vi "treadmill_main.vi"() -> ()   [LabVIEW 2019]
uses:
  #typedef_DefinedStates.ctl
  OperateCluster.ctl
  SpeedAndTimeCluster.ctl
  FollowingSteps.ctl
panel:
  out "Speed":u16
  out "Time":dbl
  in  "Slower":bool
  in  "Faster":bool
  in  "Exit":bool
  in  "QuickStart":bool
  in  "Start Program":bool
  in  "DefineProg":bool
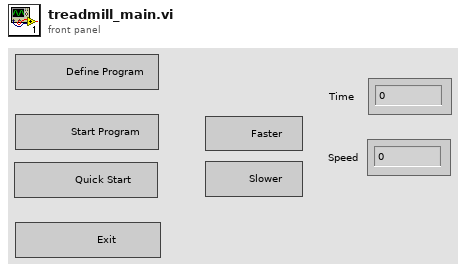
[diagram p1: front panel]
types:
  T1 = typedef "OperateCluster.ctl" = cluster{"SpeedAndTime":T2, "Following Steps":T3, "CurrentStep 2":T2, "WorkStepsCoutner":u16, "LastIndex":i32, "LastState":T4}
  T2 = typedef "SpeedAndTimeCluster.ctl" = cluster{"Time ":dbl, " Speed":u16}
  T3 = typedef "FollowingSteps.ctl" = T2[]
  T4 = typedef "#typedef_DefinedStates.ctl" = enum16{"Init", "Config", "DefineProgram", "StartProgram", "WorkAsUWant", "ChangeStep", "WorkwithSteps", "ExitProgram"}
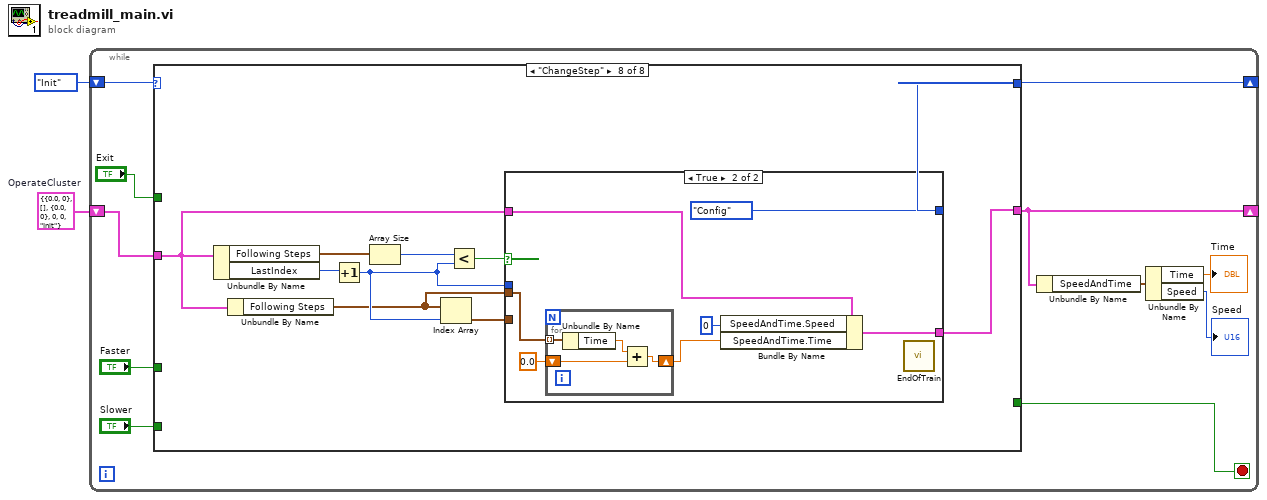
[diagram p0: block diagram]
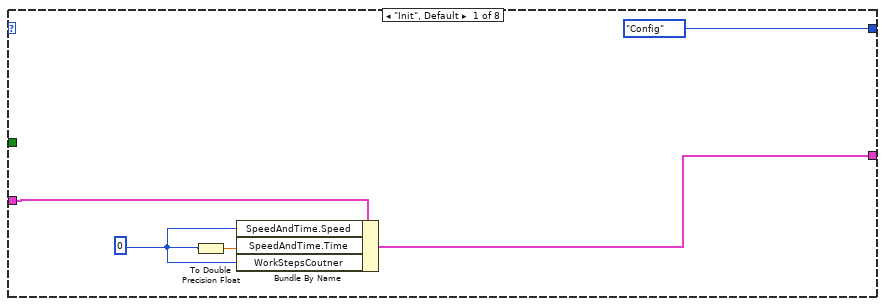
[diagram p2: hidden frame]
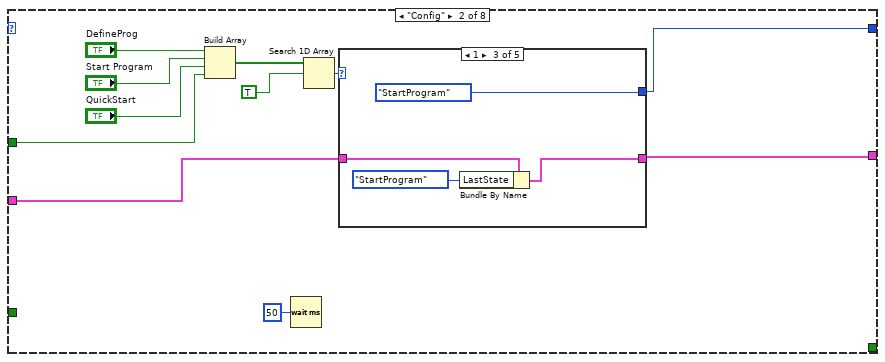
[diagram p3: hidden frame]
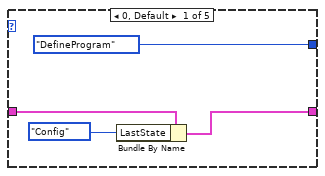
[diagram p4: hidden frame]
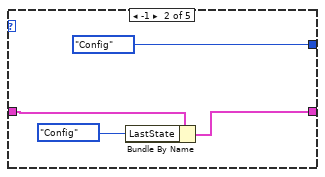
[diagram p5: hidden frame]
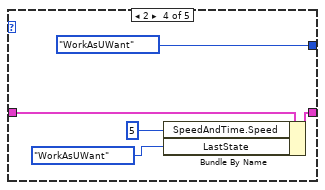
[diagram p6: hidden frame]
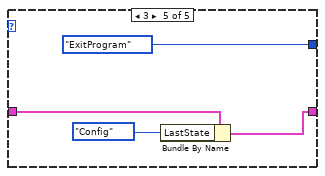
[diagram p7: hidden frame]
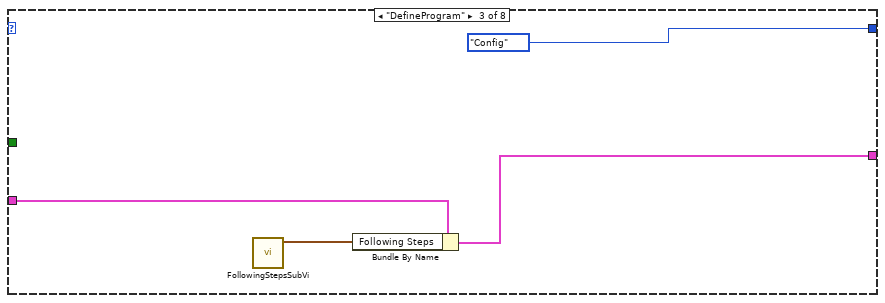
[diagram p8: hidden frame]
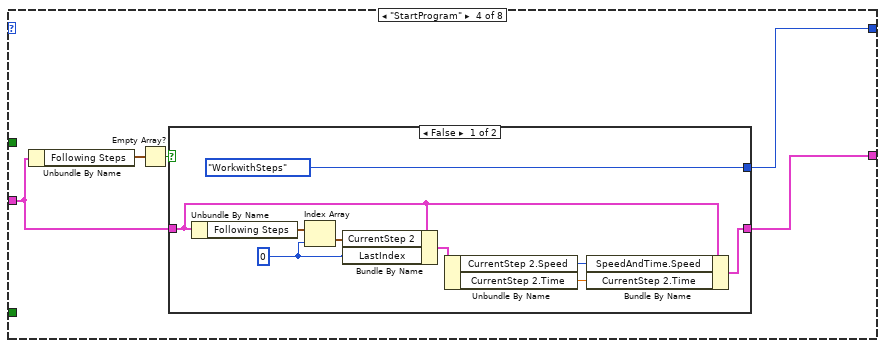
[diagram p9: hidden frame]
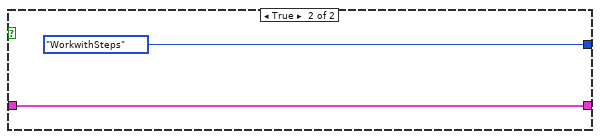
[diagram p10: hidden frame]
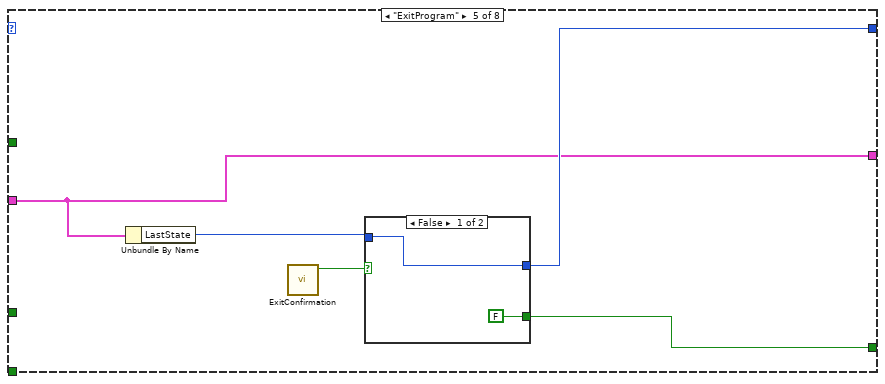
[diagram p11: hidden frame]
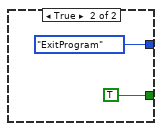
[diagram p12: hidden frame]
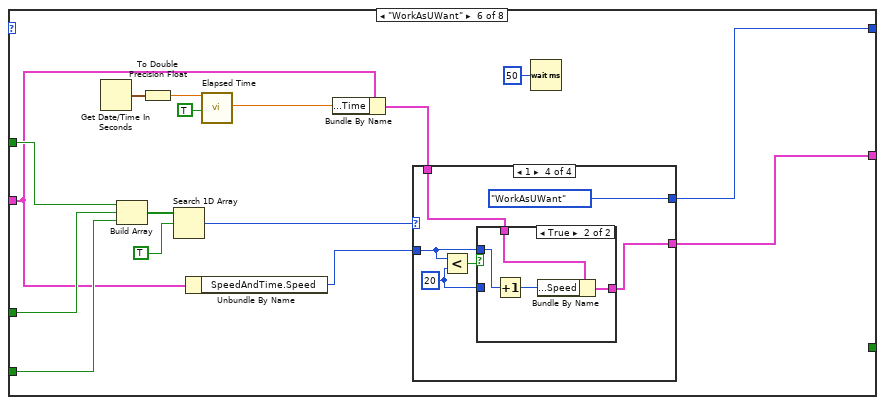
[diagram p13: hidden frame]
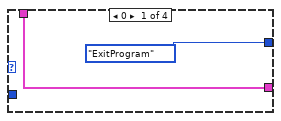
[diagram p14: hidden frame]
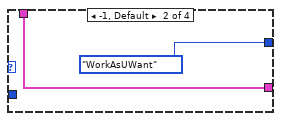
[diagram p15: hidden frame]
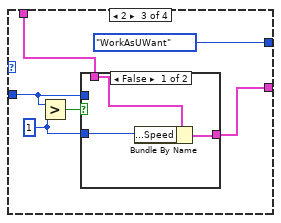
[diagram p16: hidden frame]
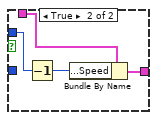
[diagram p17: hidden frame]
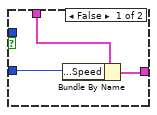
[diagram p18: hidden frame]
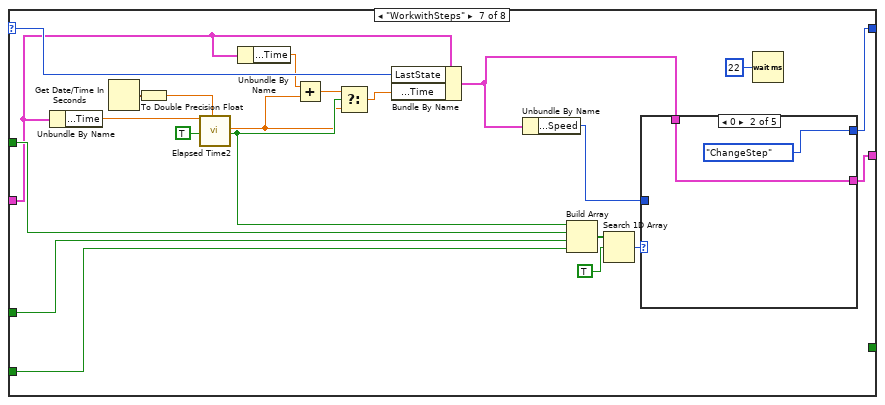
[diagram p19: hidden frame]
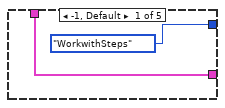
[diagram p20: hidden frame]
diagram:
  w1 = T1 {"SpeedAndTime"={"Time "=0.0, " Speed"=0}, "Following Steps"=[], "CurrentStep 2"={"Time "=0.0, " Speed"=0}, "WorkStepsCoutner"=0, "LastIndex"=0, "LastState"=enum."Init"}  # OperateCluster
  n1 = while {
    shift-right: [w11] -> _
    shift-left: #typedef_DefinedStates."Init" -> [w3]
    shift-right: [w9] -> _
    shift-left: w1 -> [w10]
    stop <- w4 stop-if-true
    n2 = case shown="\"ChangeStep\"" w3 {
      selector: w3 -> [_ _ _ _ _ _ w137 _]
      tunnel: [#typedef_DefinedStates."Config" w21 #typedef_DefinedStates."Config" w57 w74 w89 w138 w181] -> w11
      tunnel: w10 -> [w17 w24 w52 w56 w72 w86 w131 w184]
      tunnel: [w16 w23 w51 w55 w72 w88 w139 w186] -> w9
      tunnel: "Faster" -> [_ _ _ _ _ w95 w143 _]
      tunnel: "Slower" -> [_ _ _ _ _ w94 w144 _]
      tunnel: "Exit" -> [_ w20 _ _ _ w90 w142 _]
      tunnel: [_ _ _ _ w73 _ _ _] -> w4
      frame "Init", Default {
        w14 = u16 0 ("index")
        n3 = To Double Precision Float(number=w14) -> (double precision float=w15:dbl)
        n4 = Bundle By Name(cluster=w17, "SpeedAndTime.Speed"=w14, "SpeedAndTime.Time"=w15, "WorkStepsCoutner"=w14) -> (w16:T1)
      }
      frame "Config" {
        n5 = Build Array("DefineProg", "Start Program", "QuickStart", w20) -> (w26:bool[])
        n6 = Wait (ms)(milliseconds to wait=u32 50) -> ()  [unwired: 1 out]
        n7 = Search 1D Array(1D array=w26, element=TRUE) -> (index of element=w25:i32)  [unwired: 1 in]
        n8 = case shown="1" w25 {
          tunnel: [#typedef_DefinedStates."DefineProgram" #typedef_DefinedStates."Config" #typedef_DefinedStates."StartProgram" #typedef_DefinedStates."WorkAsUWant" #typedef_DefinedStates."ExitProgram"] -> w21
          tunnel: w24 -> [w32 w35 w39 w46 w48]
          tunnel: [w31 w34 w38 w45 w47] -> w23
          frame 0, Default {
            n9 = Bundle By Name(cluster=w32, "LastState"=#typedef_DefinedStates."Config") -> (w31:T1)
          }
          frame -1 {
            n10 = Bundle By Name(cluster=w35, "LastState"=#typedef_DefinedStates."Config") -> (w34:T1)
          }
          frame 1 {
            n11 = Bundle By Name(cluster=w39, "LastState"=#typedef_DefinedStates."StartProgram") -> (w38:T1)
          }
          frame 2 {
            n12 = Bundle By Name(cluster=w46, "SpeedAndTime.Speed"=u16 5 ("CurrentStep 2. Speed"), "LastState"=#typedef_DefinedStates."WorkAsUWant") -> (w45:T1)
          }
          frame 3 {
            n13 = Bundle By Name(cluster=w48, "LastState"=#typedef_DefinedStates."Config") -> (w47:T1)
          }
        }
      }
      frame "DefineProgram" {
        n14 = call "FollowingStepsSubVi.vi"() -> ("ArrayOutput"=w53:T3)  [unwired: 11 in]
        n15 = Bundle By Name(cluster=w52, "Following Steps"=w53) -> (w51:T1)
      }
      frame "StartProgram" {
        n16 = Unbundle By Name(w56) -> ("Following Steps"=w59:T3)
        n17 = Empty Array?(array=w59) -> (empty?=w58:bool)
        n18 = case shown="False" w58 {
          tunnel: [#typedef_DefinedStates."WorkwithSteps" #typedef_DefinedStates."WorkwithSteps"] -> w57
          tunnel: w56 -> [w63 w69]
          tunnel: [w62 w69] -> w55
          frame False {
            w65 = 0 ("index")
            n19 = Unbundle By Name(w63) -> ("Following Steps"=w67:T3)
            n20 = Index Array(array=w67, index=w65) -> (element=w66:T2)
            n21 = Bundle By Name(cluster=w63, "CurrentStep 2"=w66, "LastIndex"=w65) -> (w64:T1)
            n22 = Unbundle By Name(w64) -> ("CurrentStep 2.Speed"=w61:u16, "CurrentStep 2.Time"=w60:dbl)
            n23 = Bundle By Name(cluster=w63, "SpeedAndTime.Speed"=w61, "CurrentStep 2.Time"=w60) -> (w62:T1)
          }
          frame True {
          }
        }
      }
      frame "ExitProgram" {
        n24 = Unbundle By Name(w72) -> ("LastState"=w71:T4)
        n25 = call "ExitConfirmation.vi"() -> ("Output"=w75:bool)  [unwired: 11 in]
        n26 = case shown="False" w75 {
          tunnel: [w77 #typedef_DefinedStates."ExitProgram"] -> w74
          tunnel: [FALSE TRUE] -> w73
          tunnel: w71 -> [w77 _]
          frame False {
          }
          frame True {
          }
        }
      }
      frame "WorkAsUWant" {
        n27 = Get Date/Time In Seconds() -> (seconds since 1Jan1904=w84:timestamp)
        n28 = Build Array(w90, w95, w94) -> (w93:bool[])
        n29 = To Double Precision Float(number=w84) -> (double precision float=w81:dbl)
        n30 = Search 1D Array(1D array=w93, element=TRUE) -> (index of element=w91:i32)  [unwired: 1 in]
        n31 = Unbundle By Name(w86) -> ("SpeedAndTime.Speed"=w87:u16)
        n32 = call "Elapsed Time"("Time Target (s)"=w81, "Auto Reset"=TRUE) -> ("Elapsed Time (s)"=w83:dbl)  [unwired: 10 in, 7 out]
        n33 = Bundle By Name(cluster=w86, "SpeedAndTime.Time"=w83) -> (w85:T1)
        n34 = case shown="1" w91 {
          tunnel: [#typedef_DefinedStates."ExitProgram" #typedef_DefinedStates."WorkAsUWant" #typedef_DefinedStates."WorkAsUWant" #typedef_DefinedStates."WorkAsUWant"] -> w89
          tunnel: w85 -> [w96 w98 w101 w114]
          tunnel: [w96 w98 w102 w113] -> w88
          tunnel: w87 -> [_ _ w100 w115]
          frame 0 {
          }
          frame -1, Default {
          }
          frame 2 {
            w103 = u16 1 ("y")
            n35 = Greater?(x=w100, y=w103) -> (0:w104:bool)
            n36 = case shown="False" w104 {
              tunnel: w101 -> [w108 w111]
              tunnel: w100 -> [_ w110]
              tunnel: [w106 w109] -> w102
              tunnel: w103 -> [w107 _]
              frame False {
                n37 = Bundle By Name(cluster=w108, "SpeedAndTime.Speed"=w107) -> (w106:T1)
              }
              frame True {
                n38 = Decrement(x=w110) -> (x-1=w112:u16)
                n39 = Bundle By Name(cluster=w111, "SpeedAndTime.Speed"=w112) -> (w109:T1)
              }
            }
          }
          frame 1 {
            w116 = u16 20 ("y")
            n40 = Less?(x=w115, y=w116) -> (x < y?=w117:bool)
            n41 = case shown="True" w117 {
              tunnel: w114 -> [w121 w124]
              tunnel: w115 -> [_ w123]
              tunnel: [w119 w122] -> w113
              tunnel: w116 -> [w120 _]
              frame False {
                n42 = Bundle By Name(cluster=w121, "CurrentStep 2.Speed"=w120) -> (w119:T1)
              }
              frame True {
                n43 = Increment(x=w123) -> (x+1=w125:u16)
                n44 = Bundle By Name(cluster=w124, "SpeedAndTime.Speed"=w125) -> (w122:T1)
              }
            }
          }
        }
        n45 = Wait (ms)(milliseconds to wait=u32 50) -> ()  [unwired: 1 out]
      }
      frame "WorkwithSteps" {
        n46 = Unbundle By Name(w131) -> ("CurrentStep 2.Time"=w132:dbl)
        n47 = Get Date/Time In Seconds() -> (seconds since 1Jan1904=w136:timestamp)
        n48 = To Double Precision Float(number=w136) -> (double precision float=w133:dbl)
        n49 = call "Elapsed Time2"("Time Target (s)"=w132, "Auto Reset"=TRUE, "Set Start Time (s)"=w133) -> ("Elapsed Time (s)"=w128:dbl, "Time has Elapsed"=w129:bool)  [unwired: 9 in, 6 out]
        n50 = Unbundle By Name(w131) -> ("SpeedAndTime.Time"=w130:dbl)
        n51 = Add(x=w130, y=w128) -> (x+y=w127:dbl)
        n52 = Select(t=w127, s=w129, f=w128) -> (s? t:f=w126:dbl)
        n53 = Bundle By Name(cluster=w131, "LastState"=w137, "SpeedAndTime.Time"=w126) -> (w134:T1)
        n54 = Unbundle By Name(w134) -> ("CurrentStep 2.Speed"=w140:u16)
        n55 = Build Array(w129, w142, w143, w144) -> (w147:bool[])
        n56 = Search 1D Array(1D array=w147, element=TRUE) -> (index of element=w141:i32)  [unwired: 1 in]
        n57 = case shown="0" w141 {
          tunnel: w140 -> [_ _ w154 _ w168]
          tunnel: w134 -> [w149 w151 w155 w166 w169]
          tunnel: [w149 w151 w153 w166 w167] -> w139
          tunnel: [#typedef_DefinedStates."WorkwithSteps" #typedef_DefinedStates."ChangeStep" #typedef_DefinedStates."WorkwithSteps" #typedef_DefinedStates."ExitProgram" #typedef_DefinedStates."WorkwithSteps"] -> w138
          frame -1, Default {
          }
          frame 0 {
          }
          frame 2 {
            w152 = u16 20 ("y")
            n58 = Less?(x=w154, y=w152) -> (x < y?=w156:bool)
            n59 = case shown="True" w156 {
              tunnel: w155 -> [w160 w163]
              tunnel: w154 -> [_ w162]
              tunnel: [w158 w161] -> w153
              tunnel: w152 -> [w159 _]
              frame False {
                n60 = Bundle By Name(cluster=w160, "SpeedAndTime.Speed"=w159, "CurrentStep 2.Speed"=w159) -> (w158:T1)
              }
              frame True {
                n61 = Increment(x=w162) -> (x+1=w164:u16)
                n62 = Bundle By Name(cluster=w163, "SpeedAndTime.Speed"=w164, "CurrentStep 2.Speed"=w164) -> (w161:T1)
              }
            }
          }
          frame 1 {
          }
          frame 3 {
            w171 = u16 1 ("y")
            n63 = Greater?(x=w168, y=w171) -> (0:w172:bool)
            n64 = case shown="False" w172 {
              tunnel: w169 -> [w175 w178]
              tunnel: w168 -> [_ w177]
              tunnel: [w173 w176] -> w167
              tunnel: w171 -> [w174 _]
              frame False {
                n65 = Bundle By Name(cluster=w175, "SpeedAndTime.Speed"=w174, "CurrentStep 2.Speed"=w174) -> (w173:T1)
              }
              frame True {
                n66 = Decrement(x=w177) -> (x-1=w179:u16)
                n67 = Bundle By Name(cluster=w178, "SpeedAndTime.Speed"=w179, "CurrentStep 2.Speed"=w179) -> (w176:T1)
              }
            }
          }
        }
        n68 = Wait (ms)(milliseconds to wait=u32 22) -> ()  [unwired: 1 out]
      }
      frame "ChangeStep" {
        n69 = Unbundle By Name(w184) -> ("Following Steps"=w188:T3, "LastIndex"=w189:i32)
        n70 = Unbundle By Name(w184) -> ("Following Steps"=w180:T3)
        n71 = Increment(x=w189) -> (x+1=w182:i32)
        n72 = Array Size(array=w188) -> (size(s)=w187:i32)
        n73 = Index Array(array=w180, index=w182) -> (element=w183:T2)
        n74 = Less?(x=w187, y=w182) -> (x < y?=w185:bool)
        n75 = case shown="True" w185 {
          tunnel: [w191 w201] -> w186
          tunnel: w184 -> [w197 w203]
          tunnel: w183 -> [w196 _]
          tunnel: w182 -> [w195 _]
          tunnel: [#typedef_DefinedStates."WorkwithSteps" #typedef_DefinedStates."Config"] -> w181
          tunnel: w180 -> [_ w200]
          frame False {
            n76 = Bundle By Name(cluster=w197, "LastIndex"=w195, "CurrentStep 2"=w196) -> (w193:T1)
            n77 = Unbundle By Name(w193) -> ("CurrentStep 2.Speed"=w192:u16, "CurrentStep 2.Time"=w190:dbl)
            n78 = Bundle By Name(cluster=w193, "SpeedAndTime.Speed"=w192, "CurrentStep 2.Time"=w190) -> (w191:T1)
          }
          frame True {
            n79 = for {
              tunnel: w200 -> [w208] mode=indexing
              shift-right: [w206] -> w198
              shift-left: 0.0 -> [w205]
              n80 = Unbundle By Name(w208) -> ("Time"=w207:dbl)
              n81 = Add(x=w207, y=w205) -> (x+y=w206:dbl)
            }
            n82 = Bundle By Name(cluster=w203, "SpeedAndTime.Speed"=u16 0 ("SpeedAndTime. Speed"), "SpeedAndTime.Time"=w198) -> (w201:T1)
            n83 = call "EndOfTrain.vi"() -> ()  [unwired: 12 in]
          }
        }
      }
    }
    n84 = Unbundle By Name(w9) -> ("SpeedAndTime"=w8:T2)
    n85 = Unbundle By Name(w8) -> ("Time"=→"Time":dbl, "Speed"=→"Speed":u16)
  }
